vi "Ignore_Channel_evaluate.vi"(4 "Column Index":i32, 5 "Ignore When String":string, 6 "Template Names":string[](array[string]), 7 "Data":string[][](array[string])) -> (3 "Data Out":string[][](array[string]))   [LabVIEW 2013]
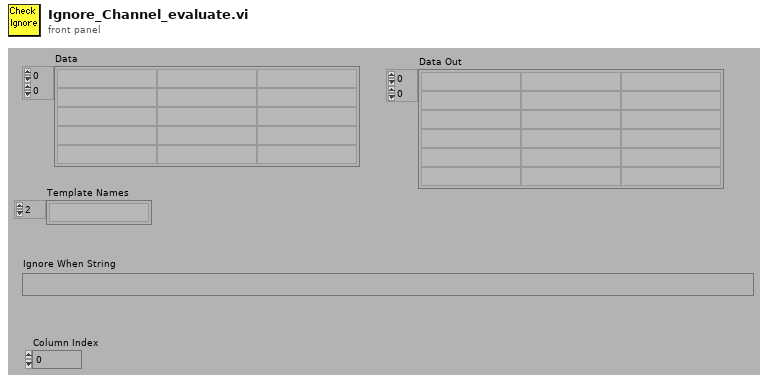
[diagram p1: front panel]
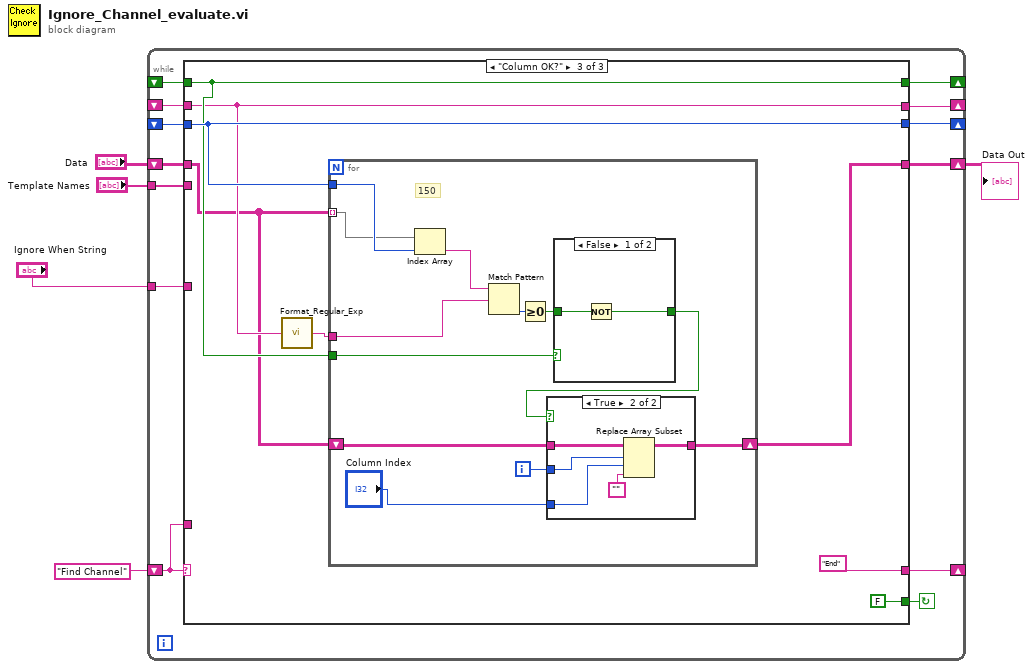
[diagram p0: block diagram]
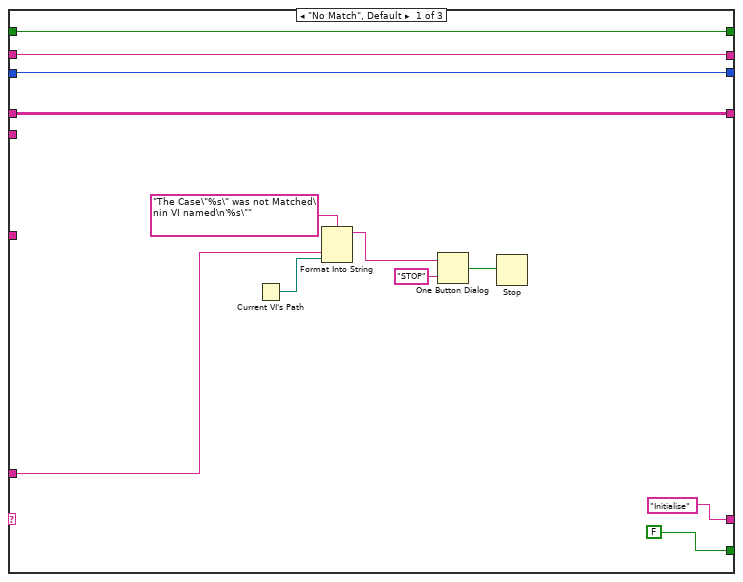
[diagram p2: hidden frame]
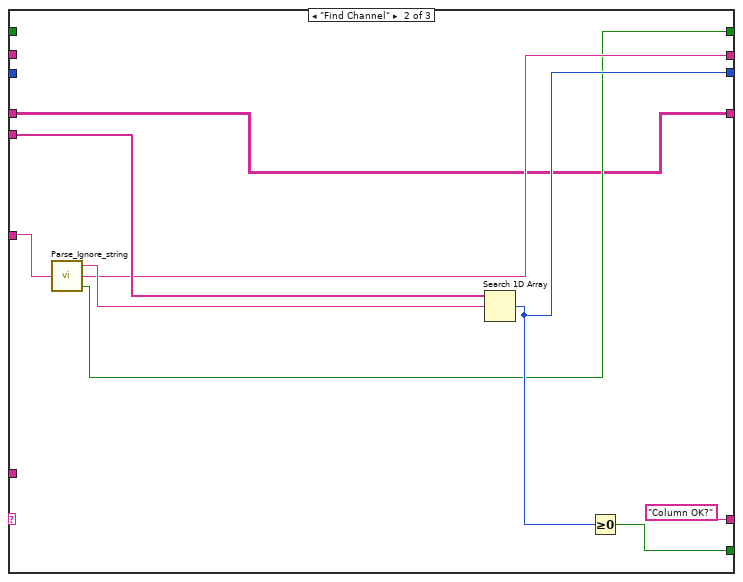
[diagram p3: hidden frame]
diagram:
  n1 = while {
    shift-left: _ -> [w13]
    shift-right: [w14] -> _
    tunnel: "Template Names" -> [w15]
    shift-left: "Find Channel" -> [w16]
    shift-right: [w17] -> _
    tunnel: "Ignore When String" -> [w12]
    shift-right: [w11] -> _
    shift-left: _ -> [w10]
    shift-right: [w9] -> _
    shift-left: _ -> [w8]
    shift-right: [w7] -> w1
    shift-left: "Data" -> [w6]
    stop <- w18 continue-if-true
    n2 = case shown="\"Column OK?\"" w16 {
      tunnel: [FALSE w36 FALSE] -> w18
      tunnel: ["Initialise" "Column OK?" "End"] -> w17
      tunnel: w16 -> [w25 _ _]
      tunnel: w15 -> [_ w38 _]
      tunnel: [w22 w37 w45] -> w14
      tunnel: w13 -> [w22 _ w45]
      tunnel: w12 -> [_ w32 _]
      tunnel: [w20 w34 w42] -> w11
      tunnel: w10 -> [w20 _ w42]
      tunnel: [w21 w33 w43] -> w9
      tunnel: w8 -> [w21 _ w43]
      tunnel: [w19 w31 w40] -> w7
      tunnel: w6 -> [w19 w31 w41]
      frame "No Match", Default {
        n3 = Current VI's Path() -> (path=w24:path)
        n4 = Format Into String(format string="The Case\"%s\" was not Matched\nin VI named\n'%s\"" ("Format String"), w25, w24) -> (resulting string=w28:string)  [unwired: 2 in, 1 out]
        n5 = One Button Dialog(message=w28, button name ("OK")="STOP") -> (true=w26:bool)
        n6 = Stop(stop? (T)=w26) -> ()
      }
      frame "Find Channel" {
        n7 = call "Parse_Ignore_string.vi"("Ignore When String"=w32) -> ("Channel Name"=w35:string, "Search String"=w34:string, "Does Contain"=w33:bool)
        n8 = Search 1D Array(1D array=w38, element=w35) -> (index of element=w37:i32)  [unwired: 1 out]
        n9 = Greater Or Equal To 0?(x=w37) -> (x >= 0?=w36:bool)
      }
      frame "Column OK?" {
        n10 = call "Format_Regular_Exp.vi"("Regular expression"=w42) -> ("Case Insensitive for html"=w46:string)
        n11 = for {
          tunnel: w41 -> [w56] mode=indexing
          tunnel: w45 -> [w57]
          tunnel: w46 -> [w59]
          tunnel: w43 -> [w58]
          shift-right: [w48] -> w40
          shift-left: w41 -> [w49]
          i -> [w52]
          # "150"
          n12 = Index Array(array=w56, index=w57) -> (element=w55:string)
          n13 = Match Pattern(string=w55, regular expression=w59) -> (offset past match=w54:i32)  [unwired: 4 out]
          n14 = Greater Or Equal To 0?(x=w54) -> (x >= 0?=w53:bool)
          n15 = case shown="False" w58 {
            tunnel: [w66 w68] -> w50
            tunnel: w53 -> [w67 w68]
            frame False {
              n16 = Not(x=w67) -> (.not. x?=w66:bool)
            }
            frame True {
            }
          }
          n17 = case shown="True" w50 {
            tunnel: w49 -> [w60 w65]
            tunnel: w52 -> [_ w62]
            tunnel: [w60 w64] -> w48
            tunnel: "Column Index" -> [_ w61]
            frame False {
            }
            frame True {
              n18 = Replace Array Subset(array=w65, new element="", index (row)=w62, index (col)=w61) -> (w64:string[][])
            }
          }
        }
      }
    }
  }
  "Data Out" <- w1
